vi "Initialize Plugin.vi"(7 "component name":string, 8 "error in":errorcluster, 10 "Plugin Configuration":refnum<class "Plugin Configuration.lvclass">, 11 "RDMA Transceiver in":refnum<class "RDMA Transceiver.lvclass">) -> (0 "error out":errorcluster, 3 "RDMA Transceiver out":refnum<class "RDMA Transceiver.lvclass">)   [LabVIEW 2021, in "RDMA.lvlib" / "RDMA Transceiver.lvclass"]
doc: "Initializes all transfer groups"
uses:
  RDMA Transceiver.lvclass
  DSF Core.lvlibp/Classes/Configuration/Core/Plugin/Plugin Configuration.lvclass
  C:/Git/fmussi_niveristand-data-sharing-framework-custom-device-plugins/Components/DSF Core.lvlibp/Classes/Configuration/Core/Core Configuration.lvclass
  Configuration/Plugin/RDMA Plugin Configuration.lvclass
  RDMA Transceiver.lvclass/RDMA Transceiver.ctl
  DSF Core.lvlibp/Classes/Configuration/Core/Core Configuration.lvclass
  Debug/VsDebugLibrary.lvlib
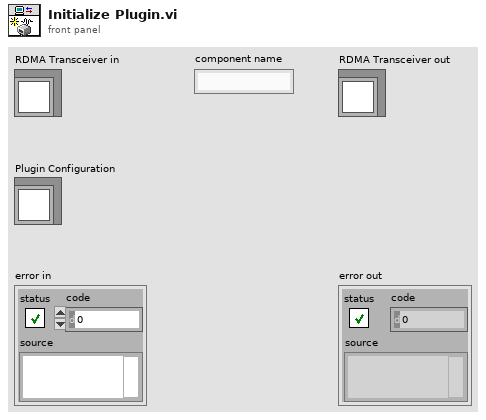
[diagram p1: front panel]
types:
  T1 = typedef "DSF Core.lvlibp/DSF Settings Info.ctl" = cluster{"component":string, "values":cluster{"key":string, "value":string}[]}
  T2 = typedef "RDMA.lvlib/RDMA Plugin Configuration.lvclass/Plugin Settings.ctl" = cluster{"initialization timeout s":dbl}
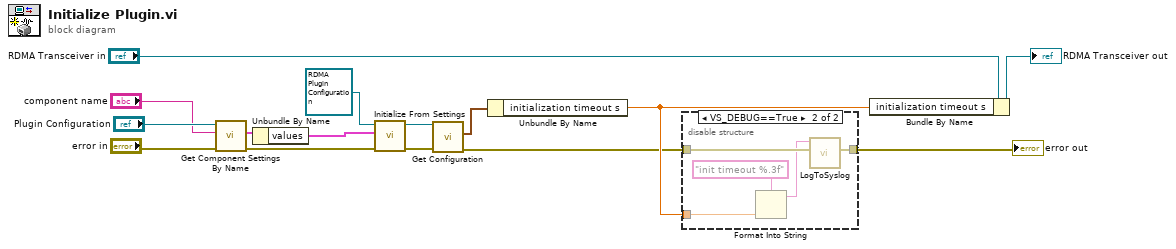
[diagram p0: block diagram]
diagram:
  n1 = call "Get Component Settings By Name.vi"("error in (no error)"="error in", "component name"="component name", "Runtime Configuration in"="Plugin Configuration") -> ("error out"=w7:errorcluster, "component settings"=w9:T1)  [unwired: 6 in, 1 out]
  n2 = Unbundle By Name(w9) -> ("values"=w8:cluster{"key":string, "value":string}[])
  n3 = call-dynamic "Initialize From Settings.vi"("error in (no error)"=w7, "settings"=w8, "RDMA Plugin Configuration in"=refnum<class "RDMA Plugin Configuration.lvclass"> refnum ("RDMA.lvlib:RDMA Plugin Configuration.lvclass")) -> ("error out"=w5:errorcluster, "RDMA Plugin Configuration out"=w6:refnum<class "RDMA Plugin Configuration.lvclass">)  [unwired: 7 in]
  n4 = call "Get Configuration.vi"("error in (no error)"=w5, "RDMA Plugin Configuration in"=w6) -> ("error out"=w2:errorcluster, "plugin settings"=w4:T2)  [unwired: 7 in, 1 out]
  n5 = Unbundle By Name(w4) -> ("initialization timeout s"=w3:dbl)
  n6 = disable-structure shown="VS_DEBUG==True" {
    disable-tunnel: w3 -> [_ w19]
    disable-tunnel: w2 -> [w16 w21]
    disable-tunnel: [w16 w20] -> w1
    frame condition #0 (active) {
    }
    frame condition #1 {
      n7 = Format Into String(format string="init timeout %.3f", w19) -> (resulting string=w18:string)  [unwired: 2 in, 1 out]
      n8 = call "LogToSyslog.vi"("error in (no error)"=w21, "message"=w18) -> ("error out"=w20:errorcluster)  [unwired: 8 in, 1 out]
    }
  }
  "error out" <- w1
  n9 = Bundle By Name(cluster="RDMA Transceiver in", "initialization timeout s"=w3) -> (→"RDMA Transceiver out":refnum<class "RDMA Transceiver.lvclass">)
